vi "cell_values.vi"(2 "Voltage in":cluster{"Voltage":dbl, dbl}[](array[cluster]), 3 "lower limit":i32, 4 "Voltage":dbl, 5 "Voltage ID":i32, 6 "upper limit":i32) -> (0 "Voltage Out":cluster{"Voltage":dbl, dbl}[](array[cluster]))   [LabVIEW 2017]
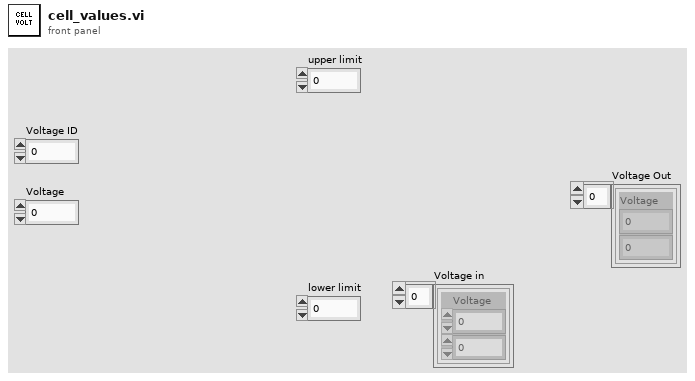
[diagram p1: front panel]
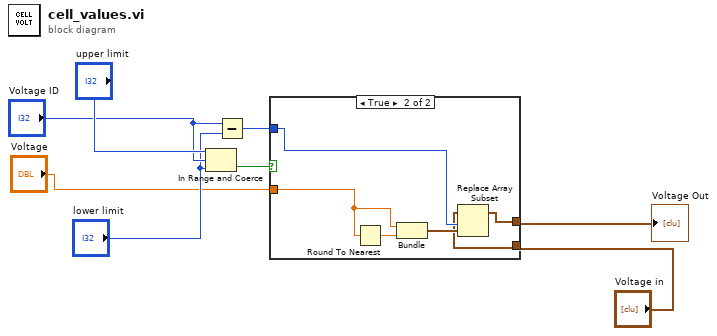
[diagram p0: block diagram]
diagram:
  n1 = In Range and Coerce(upper limit="upper limit", x="Voltage ID", lower limit="lower limit") -> (In Range?=w3:bool)  [unwired: 1 out]
  n2 = Subtract(x="Voltage ID", y="lower limit") -> (x-y=w2:i32)
  n3 = case shown="True" w3 {
    tunnel: "Voltage" -> [_ w14]
    tunnel: w2 -> [_ w12]
    tunnel: [w9 w11] -> w1
    tunnel: "Voltage in" -> [w9 w10]
    frame False {
    }
    frame True {
      n4 = Round To Nearest(number=w14) -> (nearest integer value=w15:dbl)
      n5 = Bundle("Voltage"=w14, w15) -> (w13:cluster{"Voltage":dbl, dbl})  [unwired: 1 in]
      n6 = Replace Array Subset(array=w10, new element=w13, index=w12) -> (w11:cluster{"Voltage":dbl, dbl}[])
    }
  }
  "Voltage Out" <- w1
